vi "RTS Client Server Data Check.vi"(4 "Skip Data Send":bool, 6 "error in (no error)":errorcluster, 7 "TCP Command":string, 8 "error IO":errorcluster, 10 "Send Data":string[][](array[string]), 11 "TCP Network Connection in":refnum<k5>) -> (0 "error out":errorcluster, 1 "Boolean":bool, 2 "data out":string, 3 "TCP Network Connection out":refnum<k5>)   [LabVIEW 2016]
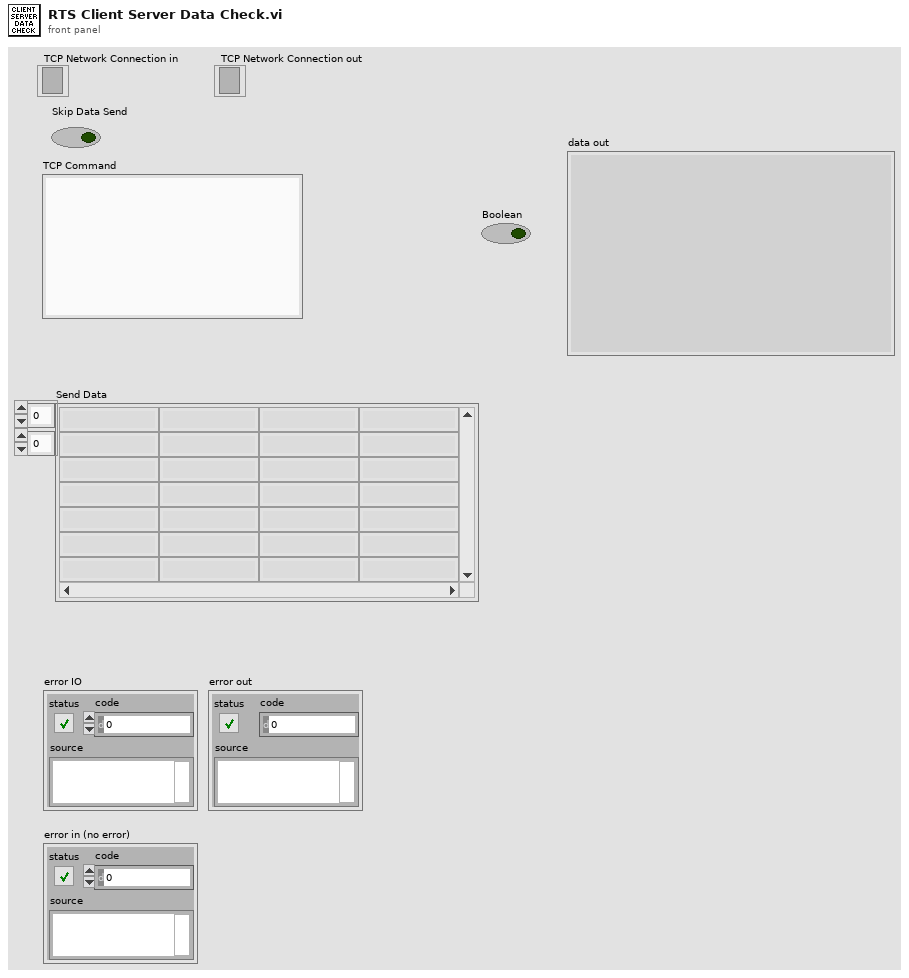
[diagram p1: front panel]
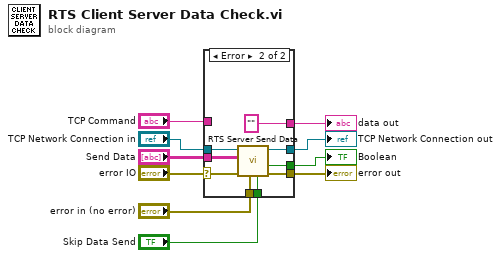
[diagram p0: block diagram]
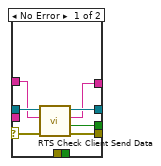
[diagram p2: hidden frame]
diagram:
  n1 = case shown="Error" "error IO" {
    selector: "error IO" -> [w16 w20]
    tunnel: "TCP Network Connection in" -> [w17 w25]
    tunnel: [w14 w24] -> w7
    tunnel: [w11 w19] -> w5
    tunnel: [w15 w26] -> w6
    tunnel: "error in (no error)" -> [_ w21]
    tunnel: [w13 "" ("data out")] -> w9
    tunnel: "TCP Command" -> [w12 _]
    tunnel: "Send Data" -> [_ w22]
    tunnel: "Skip Data Send" -> [_ w18]
    frame No Error {
      # "If the client sent data, it is saying that the connection should be closed."
      n2 = call "RTS Check Client Send Data.vi"("error in (no error)"=w16, "TCP Command"=w12, "TCP Network Connection in"=w17) -> ("error out"=w15:errorcluster, "Boolean"=w11:bool, "data out"=w13:string, "TCP Network Connection out"=w14:refnum<k5>)  [unwired: 5 in]
    }
    frame Error {
      # "Ignore connection closed and timeout errors"
      n3 = call "RTS Server Send Data.vi"("Skip Data Send"=w18, "error in (no error)"=w21, "error IO"=w20, "Send Data"=w22, "TCP Network Connection in"=w25) -> ("error out"=w26:errorcluster, "Boolean"=w19:bool, "TCP Network Connection out"=w24:refnum<k5>)  [unwired: 4 in]
    }
  }
  "data out" <- w9
  "TCP Network Connection out" <- w7
  "error out" <- w6
  "Boolean" <- w5
